vi "SRV_Queue_Get Queue Status.vi"(0 "Command-Data Queue":refnum<queue>, 11 "error in (no error)":errorcluster) -> (4 "Command-Data Queue out":refnum<queue>, 8 "# elements in queue":i32, 10 "Overflow Indicator":bool, 15 "error out":errorcluster)   [LabVIEW 2009]
uses:
  SRV_Command-Data Queue Data Type.ctl
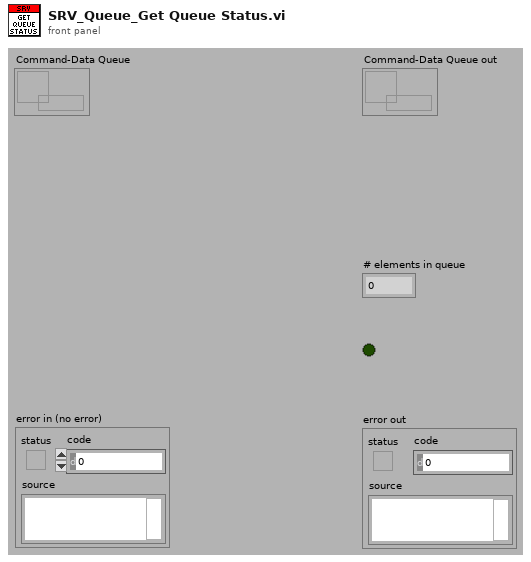
[diagram p1: front panel]
types:
  T1 = typedef "SRV_Command-Data Queue Data Type.ctl" = cluster{"Command":string, "Data":variant}
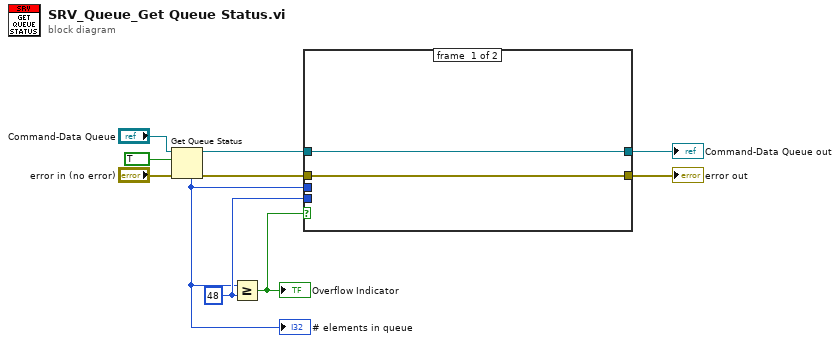
[diagram p0: block diagram]
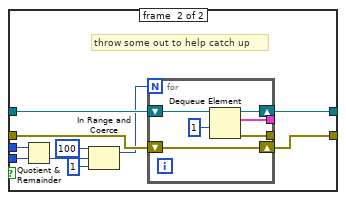
[diagram p2: hidden frame]
diagram:
  w2 = 48 ("y")
  n1 = Get Queue Status(queue="Command-Data Queue", return elements? (F)=TRUE ("return elements? (T)"), error in (no error)="error in (no error)") -> (queue out=w7:refnum<queue>, error out=w6:errorcluster, # elements in queue=w1:i32)  [unwired: 5 out]
  "# elements in queue" <- w1
  n2 = Greater Or Equal?(x=w1, y=w2) -> (x >= y?=w3:bool)
  "Overflow Indicator" <- w3
  n3 = case shown="True" w3 {
    tunnel: w7 -> [w12 w22]
    tunnel: w6 -> [w11 w21]
    tunnel: [w12 w20] -> w5
    tunnel: [w11 w19] -> w4
    tunnel: w2 -> [_ w18]
    tunnel: w1 -> [_ w17]
    frame #0 {
    }
    frame #1 {
      # "throw some out to help catch up"
      n4 = Quotient & Remainder(x=w17, y=w18) -> (floor(x/y)=w16:i32)  [unwired: 1 out]
      n5 = In Range and Coerce(upper limit=100, x=w16, lower limit=1) -> (coerced(x)=w13:i32)  [unwired: 1 out]
      n6 = for {
        N: w13 -> [_]
        tunnel: [w26] -> _
        shift-right: [w27] -> w20
        shift-left: w22 -> [w28]
        shift-right: [w24] -> w19
        shift-left: w21 -> [w24]
        tunnel: [w23] -> _
        n7 = Dequeue Element(queue=w28, timeout in ms (-1)=1) -> (queue out=w27:refnum<queue>, element=w26:T1, error out=w23:errorcluster)  [unwired: 1 in, 1 out]
      }
    }
  }
  "Command-Data Queue out" <- w5
  "error out" <- w4
